vi "Stop Core.vi"(10 "最终错误代码":i32, 11 "Beta输入":refnum<class "Map.lvclass">) -> (3 "Beta输出":refnum<class "Map.lvclass">)   [LabVIEW 2014, in "Map.lvlib" / "Map.lvclass"]
doc: "对于操作者运行过程中创建的所有并行进程，在重写Stop Core.vi的VI中应调用必要代码使其停止运行。需要停止的进程包括该操作本身创建的层层嵌套的操作者，以及所有其他异步运行的VI，比如时间延迟消息。需要停止的进程可能还包括Actor Core中的所有并行循环。（另一种方法，是在Actor Core程序框图上，在“调用父节点”结束时触发一个局部信号来停止这些进程。）\n\n<b>最终错误代码</b>输入表示操作者退出时设定的错误。0表示无错误。该错误代码可用于区分“正常停止”和“紧急停止”，从而向其他操作者发送信号。一般用非零值表示“紧急停止”，当然对于某个特定的操作者也可采用其他的表示方法。请注意，1608是个特殊的错误代码，表示当前操作者本身被“紧急停止”，如出现该错误，只能直接传递该代码。"
uses:
  Map.lvclass
  Wrapper_lib/zsActor/ActorWrapper.lvclass
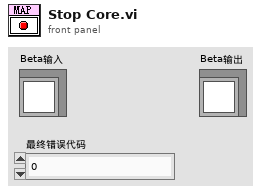
[diagram p1: front panel]
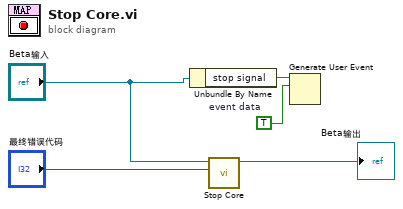
[diagram p0: block diagram]
diagram:
  w3 = TRUE  # event data
  n1 = Unbundle By Name("Beta输入") -> ("stop signal"=w2:refnum<user-event>)
  n2 = call-parent "Stop Core.vi"("final error code"="最终错误代码", "Actor in"="Beta输入") -> ("Actor out"=→"Beta输出":refnum<class "Map.lvclass">)  [unwired: 9 in]
  n3 = Generate User Event(user event=w2, event data cluster=w3) -> ()  [unwired: 2 in, 2 out]
